vi "Source Amplitude.vi"(0 "VISA resource name":refnum<visa-resource-name>="GPIB0::24::INSTR", 1 "Source Function":enum16{"CURR", "VOLT"}(ring)=enum."VOLT", 2 "Mode":enum16{"IMM", "TRIGGERED"}(ring)=enum."TRIGGERED", 3 "Source Level":dbl=10.0, 11 "error in (no error)":errorcluster) -> (4 "VISA resource name out":refnum<visa-resource-name>="GPIB0::24::INSTR", 15 "error out":errorcluster)   [LabVIEW 2010]
doc: "This Vi allows user to set up the basic source functions. Such as type, level, range, and delay. The VI can be modified to configure other aspects of source."
uses:
  <instrlib>/Keithley 24XX/Keithley 24XX.lvlib
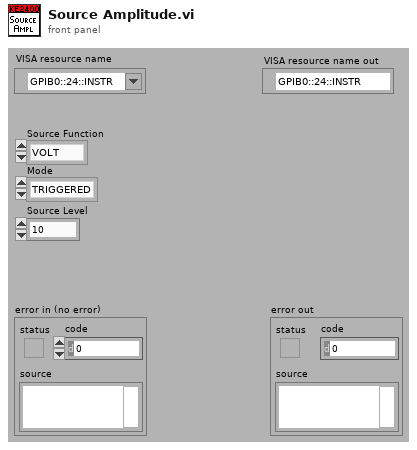
[diagram p1: front panel]
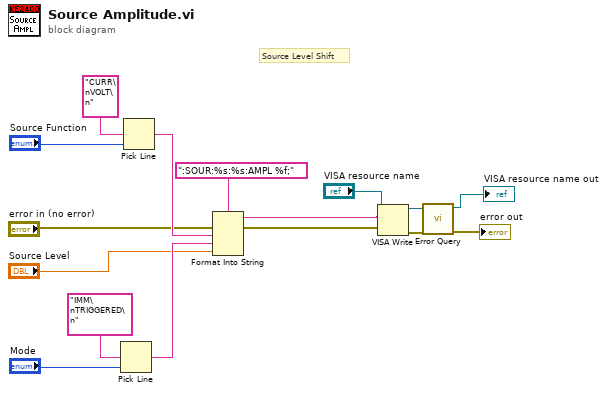
[diagram p0: block diagram]
diagram:
  # "Source Level Shift"
  n1 = Pick Line(multi-line string="IMM\nTRIGGERED\n", line index="Mode") -> (output string=w6:string)  [unwired: 1 out]
  n2 = Pick Line(multi-line string="CURR\nVOLT\n", line index="Source Function") -> (output string=w13:string)  [unwired: 1 out]
  n3 = Format Into String(format string=":SOUR:%s:%s:AMPL %f;", error in="error in (no error)", w13, w6, "Source Level") -> (resulting string=w10:string, error out=w9:errorcluster)  [unwired: 1 in]
  n4 = VISA Write(VISA resource name="VISA resource name", write buffer=w10, error in (no error)=w9) -> (VISA resource name out=w4:refnum<visa-resource-name>, error out=w3:errorcluster)  [unwired: 1 out]
  n5 = call <instrlib>:"Error Query.vi"("error in (no error)"=w3, "VISA resource name"=w4) -> ("error out"=→"error out":errorcluster, "VISA resource name out"=→"VISA resource name out":refnum<visa-resource-name>)  [unwired: 6 in, 2 out]
